vi "Get Channel List.vi"(4 "error in":errorcluster, 5 "channel names":string, 6 "group name":string, 7 "tdms file":refnum<k34>) -> (0 "error out":errorcluster, 1 "channel names out":string[](array[string]), 2 "group names out":string[](array[string]), 3 "tdms file out":refnum<k34>)   [LabVIEW 2018, in "NI_TDMS File Viewer.lvlib"]
uses:
  NI_TDMS File Viewer.lvlib
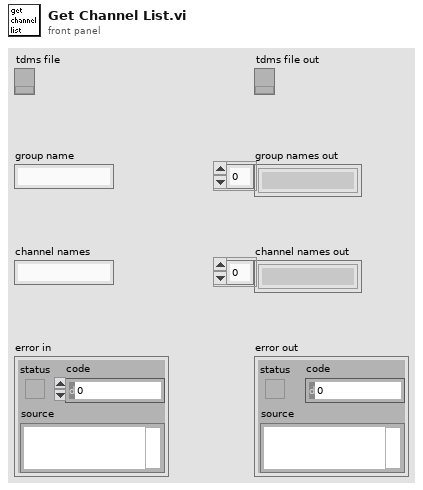
[diagram p1: front panel]
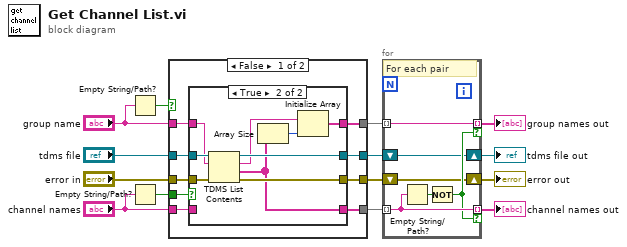
[diagram p0: block diagram]
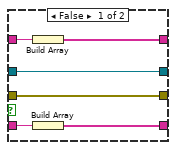
[diagram p2: hidden frame]
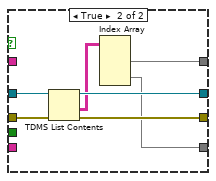
[diagram p3: hidden frame]
diagram:
  n1 = Empty String/Path?(string/path="group name") -> (empty?=w12:bool)
  n2 = Empty String/Path?(string/path="channel names") -> (empty?=w10:bool)
  n3 = case shown="False" w12 {
    tunnel: "tdms file" -> [w21 w43]
    tunnel: "error in" -> [w23 w45]
    tunnel: "channel names" -> [w20 _]
    tunnel: [w22 w44] -> w2
    tunnel: [w19 w42] -> w4
    tunnel: [w18 w41] -> w6
    tunnel: "group name" -> [w17 _]
    tunnel: [w16 w40] -> w8
    tunnel: w10 -> [w15 _]
    frame False {
      n4 = case shown="True" w15 {
        tunnel: w21 -> [w28 w36]
        tunnel: w23 -> [w29 w38]
        tunnel: [w29 w37] -> w22
        tunnel: [w28 w35] -> w19
        tunnel: w17 -> [w25 w34]
        tunnel: [w26 w30] -> w18
        tunnel: w20 -> [w27 _]
        tunnel: [w24 w31] -> w16
        frame False {
          n5 = Build Array(w25) -> (w24:string[])
          n6 = Build Array(w27) -> (w26:string[])
        }
        frame True {
          n7 = TDMS List Contents(4:w38, 6:w34, 7:w36) -> (0:w37:errorcluster, 1:w30:string[], 2:w32:string, 3:w35:refnum<k34>)
          n8 = Array Size(array=w30) -> (size(s)=w33:i32)
          n9 = Initialize Array(w32, w33) -> (w31:string[])
        }
      }
    }
    frame True {
      n10 = TDMS List Contents(4:w45, 7:w43) -> (0:w44:errorcluster, 1:w39:string[][], 3:w42:refnum<k34>)  [unwired: 1 in, 1 out]
      n11 = Index Array(array=w39) -> (element #1=w40:string[], element #2=w41:string[])  [unwired: 4 in]
    }
  }
  n12 = for {
    tunnel: w8 -> [w51] mode=indexing
    tunnel: w6 -> [w50] mode=indexing
    tunnel: [w51] -> w7 mode=indexing if=w48
    tunnel: [w50] -> w5 mode=indexing if=w48
    shift-right: [w47] -> w3
    shift-left: w4 -> [w47]
    shift-right: [w46] -> w1
    shift-left: w2 -> [w46]
    # "For each pair"
    n13 = Empty String/Path?(string/path=w50) -> (empty?=w49:bool)
    n14 = Not(x=w49) -> (.not. x?=w48:bool)
  }
  "group names out" <- w7
  "channel names out" <- w5
  "tdms file out" <- w3
  "error out" <- w1
